vi "move.vi"(8 "error in (no error)":errorcluster, 10 "SnakeGame in":refnum<class "SnakeGame.lvclass">, 11 "Snake in":refnum<class "Snake.lvclass">) -> (0 "error out":errorcluster, 2 "SnakeGame out":refnum<class "SnakeGame.lvclass">, 3 "Snake out":refnum<class "Snake.lvclass">)   [LabVIEW 2019, in "RT_Game.lvlib" / "Snake.lvclass"]
uses:
  Snake.lvclass
  SnakeGame/SnakeGame.lvclass
  Snake.lvclass/Snake.ctl
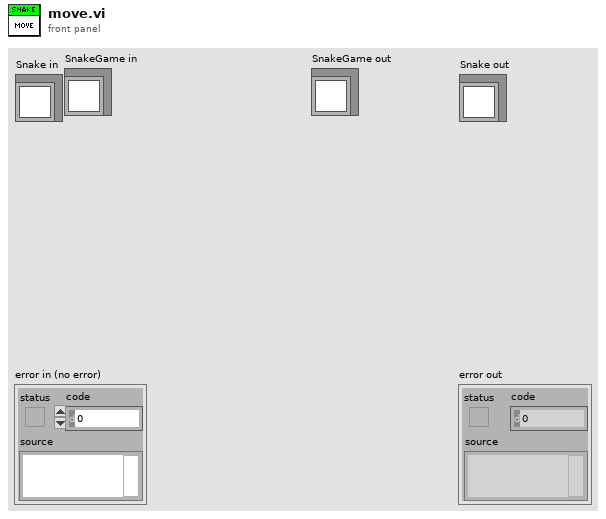
[diagram p1: front panel]
types:
  T1 = typedef "RT_Game.lvlib/Snake.lvclass/Direction.ctl" = enum16{"Up", "Left", "Down", "Right"}
  T2 = typedef "RT_Game.lvlib/Game.lvclass/Coordinate.ctl" = cluster{"x":dbl, "y":dbl}
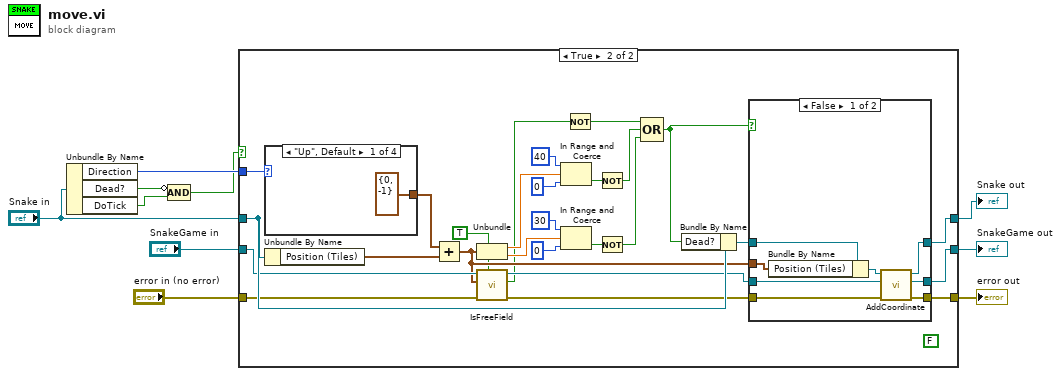
[diagram p0: block diagram]
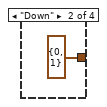
[diagram p4: hidden frame]
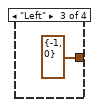
[diagram p5: hidden frame]
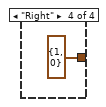
[diagram p6: hidden frame]
diagram:
  n1 = Unbundle By Name("Snake in") -> ("Direction"=w8:T1, "Dead?"=w7:bool, "DoTick"=w4:bool)
  n2 = Compound Arithmetic op=AND(invert w7, w4) -> (w5:bool)
  n3 = case shown="True" w5 {
    tunnel: "error in (no error)" -> [w12 w22]
    tunnel: [w12 w23] -> w9
    tunnel: [w13 w25] -> w3
    tunnel: "Snake in" -> [w13 w38]
    tunnel: w8 -> [_ w40]
    tunnel: [w11 w21] -> w2
    tunnel: "SnakeGame in" -> [w11 w19]
    frame False {
    }
    frame True {
      (unwired) FALSE ("x = y?")
      n4 = case shown="\"Up\", Default" w40 {
        tunnel: [cluster{"x":i8, "y":i8} {"x"=0, "y"=-1} ("x") cluster{"x":i8, "y":i8} {"x"=0, "y"=1} ("x") cluster{"x":i8, "y":i8} {"x"=-1, "y"=0} ("x") cluster{"x":i8, "y":i8} {"x"=1, "y"=0} ("x")] -> w39
        frame "Up", Default {
        }
        frame "Down" {
        }
        frame "Left" {
        }
        frame "Right" {
        }
      }
      n5 = Unbundle By Name(w38) -> ("Position (Tiles)"=w37:T2)
      n6 = Add(x=w39, y=w37) -> (x+y=w17:T2)
      n7 = Unbundle(w17) -> ("x"=w36:dbl, "y"=w33:dbl)
      n8 = call "IsFreeField.vi"("SnakesOnly?"=TRUE, "error in (no error)"=w22, "Coordinate"=w17, "SnakeGame in"=w19) -> ("error out"=w20:errorcluster, "Free?"=w16:bool, "SnakeGame out"=w18:refnum<class "SnakeGame.lvclass">)  [unwired: 5 in]
      n9 = In Range and Coerce(upper limit=i8 40, x=w36, lower limit=i8 0) -> (In Range?=w30:bool)  [unwired: 1 out]
      n10 = In Range and Coerce(upper limit=i8 30, x=w33, lower limit=i8 0) -> (In Range?=w29:bool)  [unwired: 1 out]
      n11 = Not(x=w16) -> (.not. x?=w15:bool)
      n12 = Not(x=w30) -> (.not. x?=w28:bool)
      n13 = Not(x=w29) -> (.not. x?=w27:bool)
      n14 = Compound Arithmetic op=OR(w15, w28, w27) -> (w24:bool)
      n15 = Bundle By Name(cluster=w38, "Dead?"=w24) -> (w26:refnum<class "Snake.lvclass">)
      n16 = case shown="False" w24 {
        tunnel: w26 -> [w48 w51]
        tunnel: [w45 w51] -> w25
        tunnel: w17 -> [w46 _]
        tunnel: w20 -> [w44 w50]
        tunnel: [w43 w50] -> w23
        tunnel: [w42 w49] -> w21
        tunnel: w18 -> [w41 w49]
        frame False {
          n17 = Bundle By Name(cluster=w48, "Position (Tiles)"=w46) -> (w47:refnum<class "Snake.lvclass">)
          n18 = call "AddCoordinate.vi"("error in (no error)"=w44, "SnakeGame in"=w41, "Snake in"=w47) -> ("error out"=w43:errorcluster, "SnakeGame out"=w42:refnum<class "SnakeGame.lvclass">, "Snake out"=w45:refnum<class "Snake.lvclass">)  [unwired: 6 in]
        }
        frame True {
        }
      }
    }
  }
  "error out" <- w9
  "Snake out" <- w3
  "SnakeGame out" <- w2
